vi "ShearRampStepConfigUI .vi"() -> (1 "Confirmed?":bool, 3 "ShearRampConfiguration":T1={"Rotation or Torque"="Rotation (RPM)", "Initial Value"=0.0, "Final Value"=0.0, "Step Duration"=0.0, "Number of Steps"=0, "Shear Ramp Step Array"=[], "Confirmed?"=FALSE, "Shear Step Generation"=enum."StepDurationConstant"})   [LabVIEW 2021]
uses:
  TypeDefs/ShearRampStepConfiguration.ctl
  <vilib>/Utility/file.llb/Read Delimited Spreadsheet (DBL).vi
panel:
  in  "Visualize":bool
  out "XY Graph":cluster{dbl[], "Ramp Pattern":dbl[]}(graph)
  in  "Cancel":bool
  in  "Confirm button":bool
  in  "Rotation / Torque":string(combo)="Rotation (RPM)"
  in  "Tab Control":enum32{"Constant Time", "Fill up Table"}(tab)
  in  "Initial Value":dbl
  in  "Duration":dbl caption="Step Duration (s)"
  in  "Final Value":dbl
  in  "Number of Points":i32 caption="Number of Steps"
  in  "Array - Numeric":dbl[][](array[numeric])
  in  "Import File":bool
  # "Step Value"
  # "Step Duration (s)"
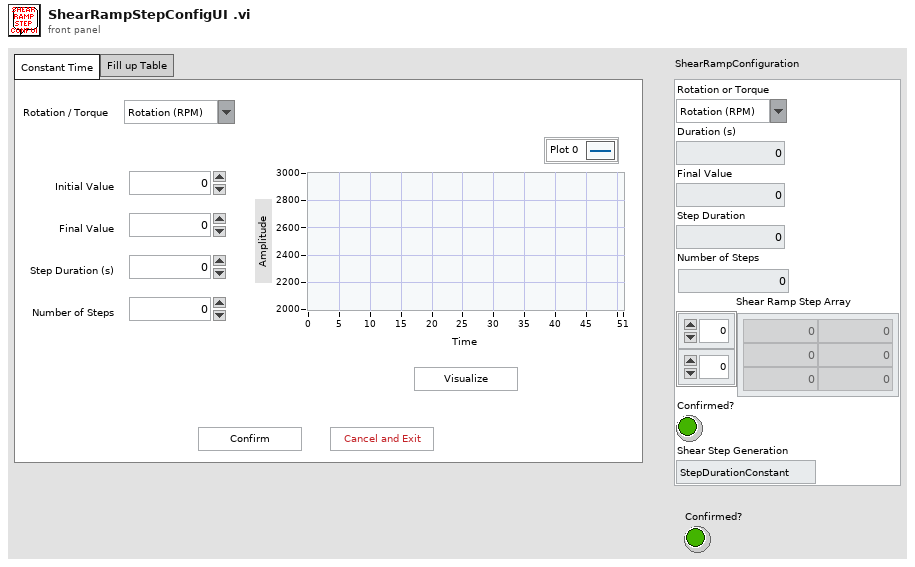
[diagram p1: front panel]
types:
  T1 = typedef "ShearRampStepConfiguration.ctl" = cluster{"Rotation or Torque":string, "Initial Value":dbl, "Final Value":dbl, "Step Duration":dbl, "Number of Steps":i32, "Shear Ramp Step Array":dbl[][], "Confirmed?":bool, "Shear Step Generation":enum16{"StepDurationConstant", "Table"}}
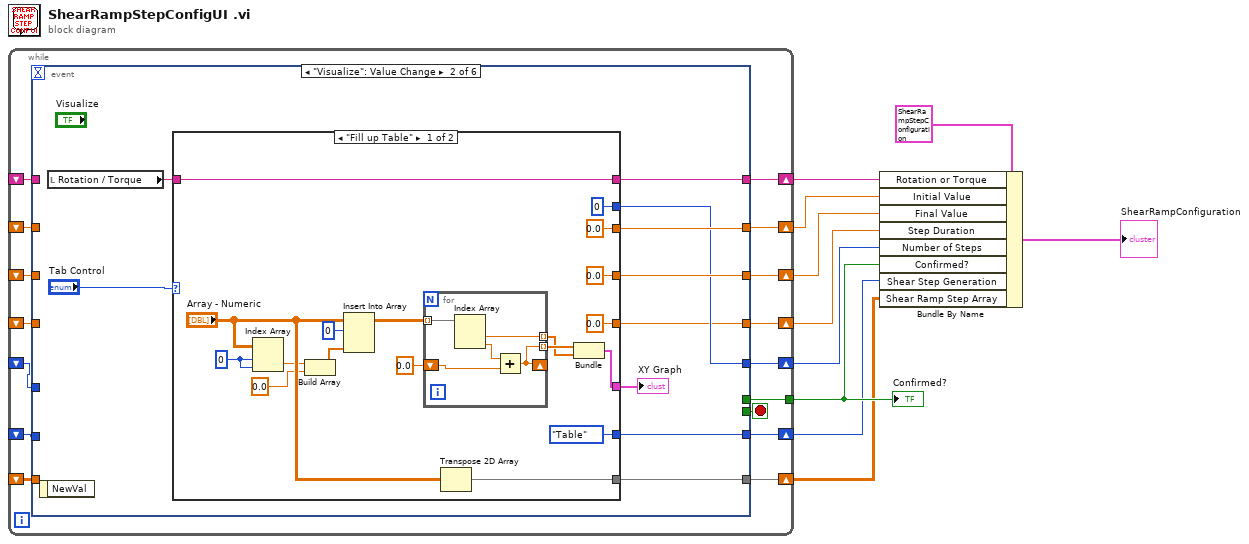
[diagram p0: block diagram]
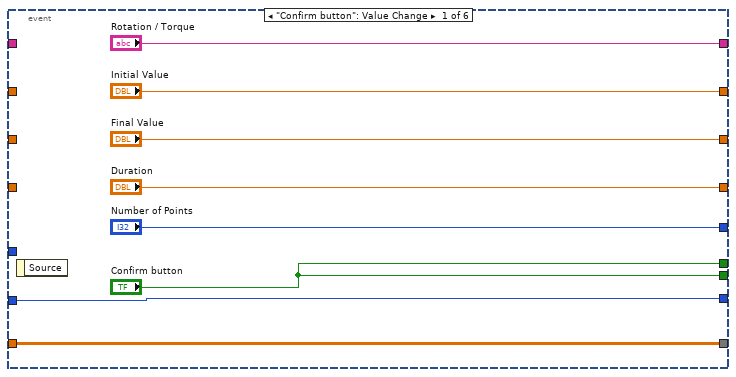
[diagram p2: hidden frame]
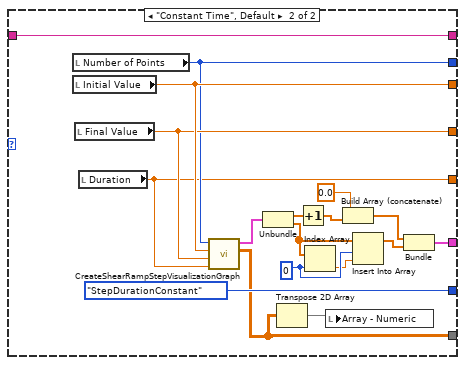
[diagram p3: hidden frame]
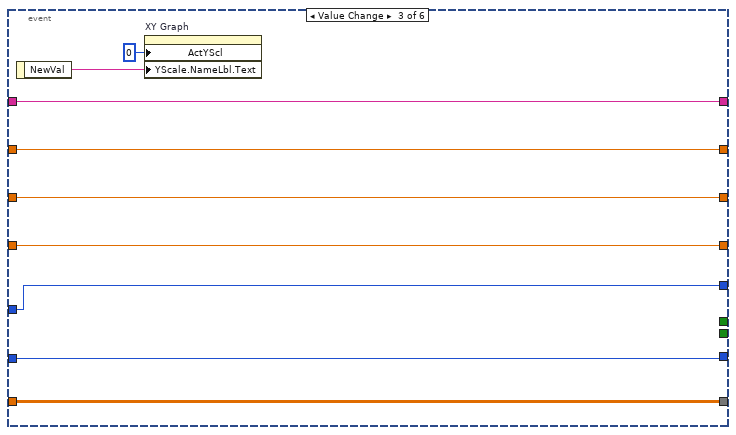
[diagram p4: hidden frame]
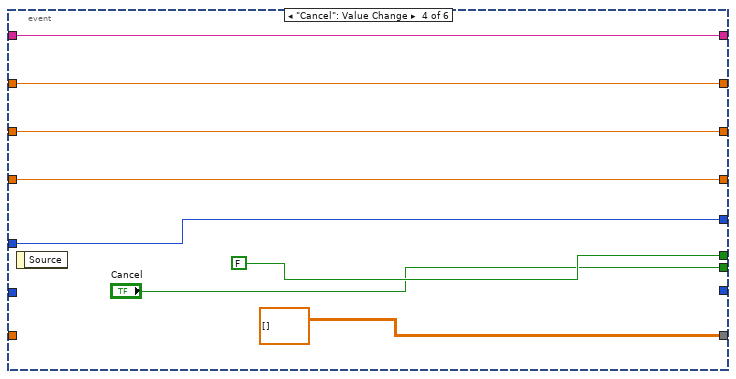
[diagram p5: hidden frame]
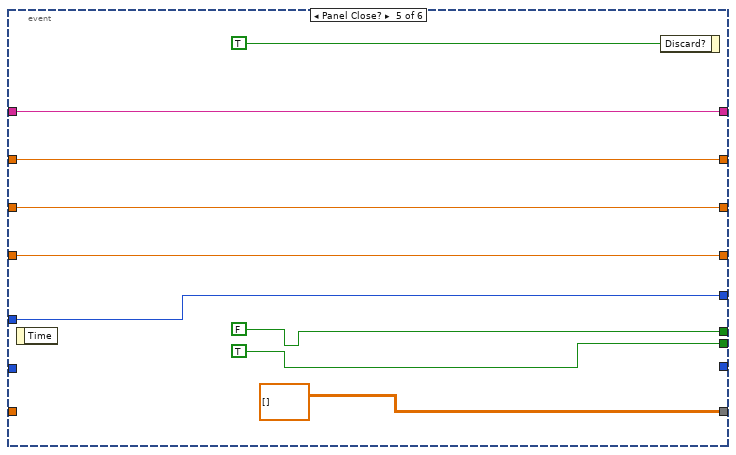
[diagram p6: hidden frame]
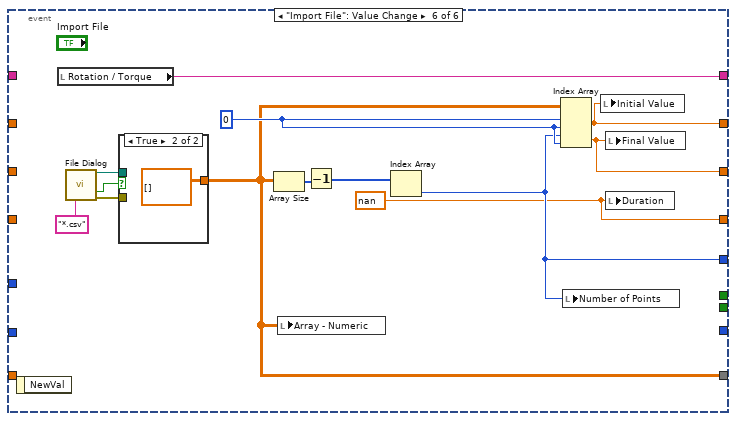
[diagram p7: hidden frame]
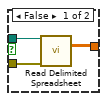
[diagram p8: hidden frame]
diagram:
  n1 = while {
    shift-right: [w26] -> w7
    shift-left: _ -> [w24]
    shift-right: [w25] -> w10
    shift-left: _ -> [w23]
    tunnel: [w22] -> w3
    shift-right: [w20] -> w6
    shift-left: _ -> [w19]
    shift-right: [w18] -> w8
    shift-left: _ -> [w17]
    shift-right: [w16] -> w5
    shift-left: _ -> [w15]
    shift-right: [w13] -> w2
    shift-left: _ -> [w12]
    shift-right: [w14] -> w1
    shift-left: _ -> [w11]
    stop <- w21 stop-if-true
    n2 = event shown="[1] \"Visualize\": Value Change" {
      selector: _ -> [_ _ _ _ _ _]
      dyn-events: _ -> [_ _ _ _ _ _]
      timeout: _ -> [_ _ _ _ _ _]
      tunnel: ["Initial Value" w44 w93 w102 w108 w115] -> w26
      tunnel: ["Rotation / Torque" w38 w94 w100 w107 w124] -> w25
      tunnel: w24 -> [_ _ w93 w102 w108 _]
      tunnel: w23 -> [_ _ w94 w100 w107 _]
      tunnel: ["Confirm button" _ _ FALSE ("Confirm button") FALSE ("Confirm button") _] -> w22
      tunnel: ["Confirm button" _ _ "Cancel" TRUE ("Cancel") _] -> w21
      tunnel: ["Duration" w40 w91 w98 w106 w112] -> w20
      tunnel: w19 -> [_ _ w91 w98 w106 _]
      tunnel: ["Final Value" w43 w92 w97 w105 w114] -> w18
      tunnel: w17 -> [_ _ w92 w97 w105 _]
      tunnel: ["Number of Points" w42 w90 w96 w104 w113] -> w16
      tunnel: w15 -> [_ _ w90 w96 w104 _]
      tunnel: [w27 w35 w88 dbl[][] [] ("Array - Numeric") dbl[][] [] ("Array - Numeric") w116] -> w14
      tunnel: [w28 w36 w89 _ _ _] -> w13
      tunnel: w12 -> [w28 _ w89 _ _ _]
      tunnel: w11 -> [w27 _ w88 _ _ _]
      event "Confirm button": Value Change {
        n3 = event-data() -> ()  [unwired: 1 in, 1 out]
      }
      event "Visualize": Value Change {
        n4 = event-data() -> ()  [unwired: 1 in, 1 out]
        n5 = local read "Rotation / Torque"() -> (w37:string)
        n6 = case shown="\"Fill up Table\"" "Tab Control" {
          tunnel: [0.0 ("Initial Value") w85] -> w44
          tunnel: [0.0 ("Final Value") w84] -> w43
          tunnel: [0 ("Number of Points") w83] -> w42
          tunnel: [w62 w70] -> w41
          tunnel: [0.0 ("Duration") w82] -> w40
          tunnel: [w61 w81] -> w38
          tunnel: w37 -> [w61 w81]
          tunnel: [enum16{"StepDurationConstant", "Table"}."Table" ("Shear Step Generation") enum16{"StepDurationConstant", "Table"}."StepDurationConstant" ("Shear Step Generation")] -> w36
          tunnel: [w45 w68] -> w35
          frame "Fill up Table" {
            w49 = 0 ("index (row)")
            n7 = Index Array(array="Array - Numeric", index (row)=w49, index (col)=w49) -> (element=w48:dbl)
            n8 = Build Array(w48, 0.0 ("element")) -> (w46:dbl[])
            n9 = Insert Into Array(array="Array - Numeric", index (row)=0, new element=w46) -> (w52:dbl[][])  [unwired: 1 in]
            n10 = for {
              tunnel: w52 -> [w67] mode=indexing
              shift-right: [w64] -> _
              shift-left: 0.0 ("Numeric") -> [w65]
              tunnel: [w64] -> w54 mode=indexing
              tunnel: [w63] -> w53 mode=indexing
              n11 = Index Array(array=w67) -> (element #1=w63:dbl, element #2=w66:dbl)  [unwired: 2 in]
              n12 = Add(x=w66, y=w65) -> (x+y=w64:dbl)
            }
            n13 = Transpose 2D Array(2D array="Array - Numeric") -> (transposed array=w45:dbl[][])
            n14 = Bundle(w54, w53) -> (w62:cluster{dbl[], dbl[]})  [unwired: 1 in]
          }
          frame "Constant Time", Default {
            w73 = 0 ("index")
            n15 = local read "Number of Points"() -> (w83:i32)
            n16 = local read "Initial Value"() -> (w85:dbl)
            n17 = local read "Final Value"() -> (w84:dbl)
            n18 = local read "Duration"() -> (w82:dbl)
            n19 = call "CreateShearRampStepVisualizationGraph.vi"("Step Duration"=w82, "Final Value"=w84, "Initial Value"=w85, "Number of Points"=w83) -> ("Shear Step Array"=w68:dbl[][], "XY Graph"=w79:cluster{dbl[], "Ramp Pattern":dbl[]})  [unwired: 6 in]
            n20 = Unbundle(w79) -> (w78:dbl[], "Ramp Pattern"=w74:dbl[])
            n21 = Transpose 2D Array(2D array=w68) -> (transposed array=w69:dbl[][])
            n22 = Increment(x=w78) -> (x+1=w75:dbl[])
            n23 = Index Array(array=w74, index=w73) -> (element=w72:dbl)
            n24 = local write "Array - Numeric"(w69) -> ()
            n25 = Build Array (concatenate)(0.0, w75) -> (w76:dbl[])
            n26 = Insert Into Array(array=w74, index=w73, new element=w72) -> (w71:dbl[])
            n27 = Bundle(w76, "Ramp Pattern"=w71) -> (w70:cluster{dbl[], "Ramp Pattern":dbl[]})  [unwired: 1 in]
          }
        }
        "XY Graph" <- w41
      }
      event Value Change {
        n28 = event-data() -> ("NewVal"=w87:string)  [unwired: 1 in]
        n29 = property on="XY Graph" class="XYGraph (strict)"("ActYScl"=0 ("Active Y Scale"), "YScale.NameLbl.Text"=w87) -> ()  [unwired: 2 in, 2 out]
      }
      event "Cancel": Value Change {
        n30 = event-data() -> ()  [unwired: 1 in, 1 out]
      }
      event Panel Close? {
        n31 = event-data() -> ()  [unwired: 1 in, 1 out]
        n32 = event-data("Discard?"=TRUE) -> ()  [unwired: 1 in, 1 out]
      }
      event "Import File": Value Change {
        w112 = nan ("Duration")
        w117 = 0 ("index (row)")
        n33 = event-data() -> ()  [unwired: 1 in, 1 out]
        n34 = local read "Rotation / Torque"() -> (w124:string)
        n35 = call "File Dialog"("pattern (all files)"="*.csv") -> ("selected path"=w122:path, "cancelled"=w120:bool, "error out"=w121:errorcluster)  [unwired: 11 in, 1 out]
        n36 = case shown="True" w120 {
          tunnel: w122 -> [w127 _]
          tunnel: w121 -> [w126 _]
          tunnel: [w125 dbl[][] [] ("all rows")] -> w116
          frame False {
            n37 = call-poly <vilib>:"Read Delimited Spreadsheet.vi"("file path (dialog if empty)"=w127, "error in (no error)"=w126) -> ("all rows"=w125:dbl[][])  [unwired: 8 in, 5 out]
          }
          frame True {
          }
        }
        n38 = Array Size(array=w116) -> (size(s)=w119:i32[])
        n39 = local write "Array - Numeric"(w116) -> ()
        n40 = Decrement(x=w119) -> (x-1=w118:i32[])
        n41 = Index Array(array=w118) -> (element=w113:i32)  [unwired: 1 in]
        n42 = Index Array(array=w116, index (row) #1=w117, index (col) #1=w117, index (row) #2=w113, index (col) #2=w117) -> (element #1=w115:dbl, element #2=w114:dbl)
        n43 = local write "Number of Points"(w113) -> ()
        n44 = local write "Initial Value"(w115) -> ()
        n45 = local write "Final Value"(w114) -> ()
        n46 = local write "Duration"(w112) -> ()
      }
    }
  }
  "Confirmed?" <- w3
  n47 = Bundle By Name(cluster=T1 {"Rotation or Torque"="Rotation (RPM)", "Initial Value"=0.0, "Final Value"=0.0, "Step Duration"=0.0, "Number of Steps"=0, "Shear Ramp Step Array"=[], "Confirmed?"=FALSE, "Shear Step Generation"=enum."StepDurationConstant"} ("ShearRampConfiguration"), "Rotation or Torque"=w10, "Initial Value"=w7, "Final Value"=w8, "Step Duration"=w6, "Number of Steps"=w5, "Confirmed?"=w3, "Shear Step Generation"=w2, "Shear Ramp Step Array"=w1) -> (→"ShearRampConfiguration":T1)
